vi "AuMT8852B EUT Supported Features Query.vi"(8 "error in (no error)":errorcluster, 11 "VISA session":refnum<visa-resource-name>) -> (0 "error out":errorcluster, 2 "error code":i32, 3 "VISA session out":refnum<visa-resource-name>, 4 "Features":T1)   [LabVIEW 2017]
doc: "Anritsu MT8852B Bluetooth Tester\n\nCauses the tester to query the EUT for a list of supported Bluetooth features.\n\nOUTPUTS\nFeatures - a breakdown of whether or not each Bluetooth feature is present in the EUT."
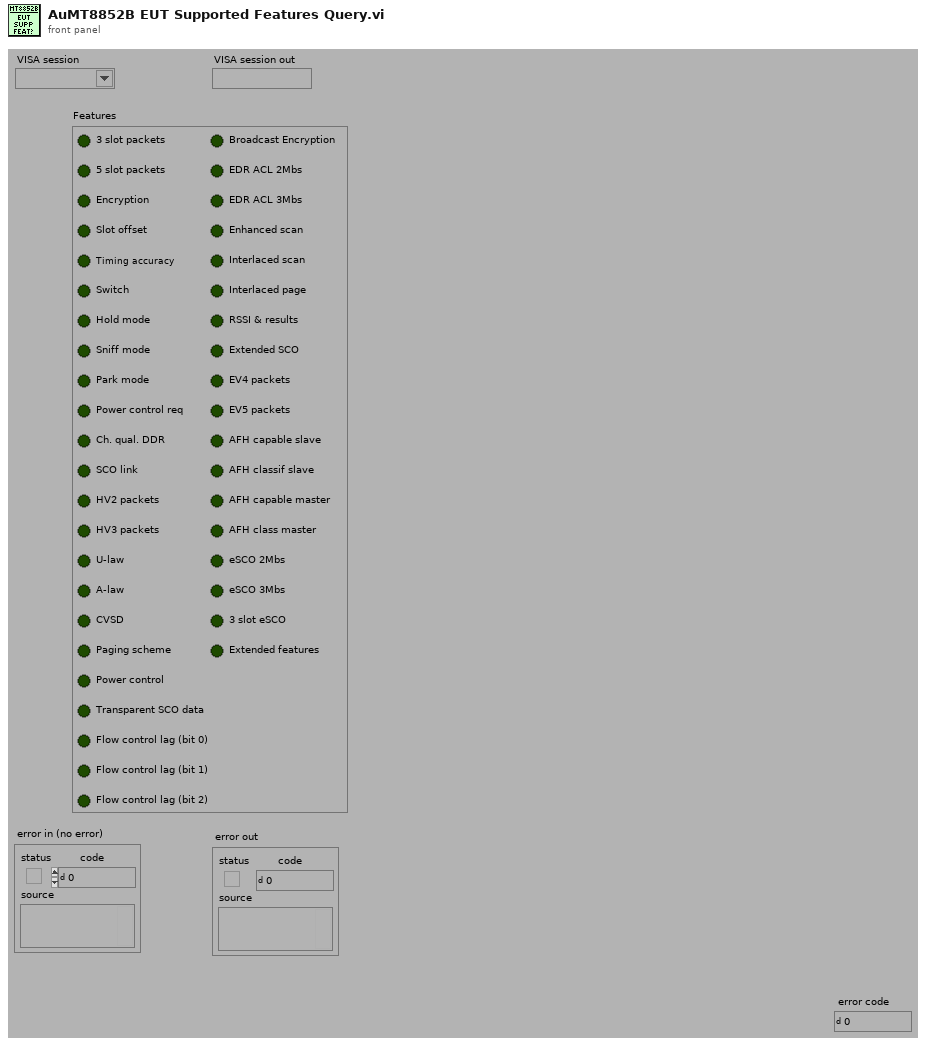
[diagram p1: front panel]
types:
  T1 = cluster{"3 slot packets":bool, "5 slot packets":bool, "Encryption":bool, "Slot offset":bool, "Timing accuracy":bool, "Switch":bool, "Hold mode":bool, "Sniff mode":bool, "Park mode":bool, "Power control req":bool, "Ch. qual. DDR":bool, "SCO link":bool, "HV2 packets":bool, "HV3 packets":bool, "U-law":bool, "A-law":bool, "CVSD":bool, "Paging scheme":bool, "Power control":bool, "Transparent SCO data":bool, "Flow control lag (bit 0)":bool, "Flow control lag (bit 1)":bool, "Flow control lag (bit 2)":bool, "Broadcast Encryption":bool, "EDR ACL 2Mbs":bool, "EDR ACL 3Mbs":bool, "Enhanced scan":bool, "Interlaced scan":bool, "Interlaced page":bool, "RSSI & results":bool, "Extended SCO":bool, "EV4 packets":bool, "EV5 packets":bool, "AFH capable slave":bool, "AFH classif slave":bool, "AFH capable master":bool, "AFH class master":bool, "eSCO 2Mbs":bool, "eSCO 3Mbs":bool, "3 slot eSCO":bool, "Extended features":bool}
  T2 = enum16{"Simulate", "Range check", "Cache", "Query instrument status"}
  T3 = cluster{"Boolean array[0]":bool, "Boolean array[1]":bool, "Boolean array[2]":bool, "Boolean array[3]":bool, "Boolean array[4]":bool, "Boolean array[5]":bool, "Boolean array[6]":bool, "Boolean array[7]":bool, "Boolean array[8]":bool, "Boolean array[9]":bool, "Boolean array[10]":bool, "Boolean array[11]":bool, "Boolean array[12]":bool, "Boolean array[13]":bool, "Boolean array[14]":bool, "Boolean array[15]":bool}
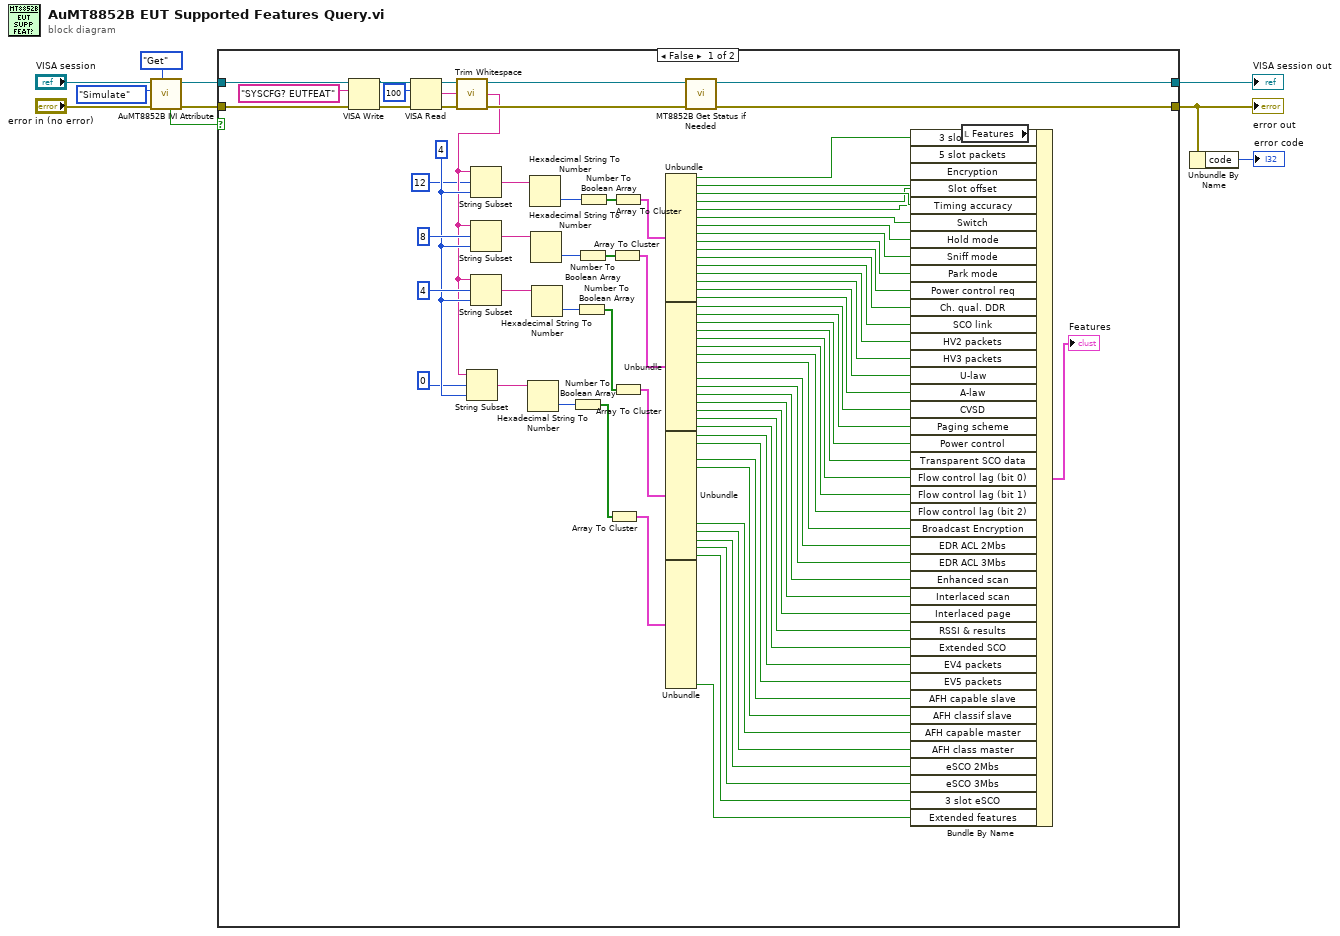
[diagram p0: block diagram]
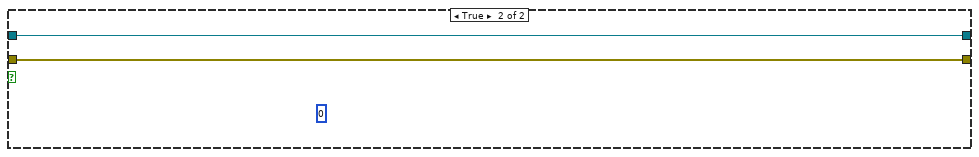
[diagram p2: hidden frame]
diagram:
  n1 = call <instrlib>:"AuMT8852B IVI Attribute.vi"("Set/Get (Set)"=enum16{"Set", "Get"}."Get", "error in (no error)"="error in (no error)", "Flag (Simulate)"=T2."Simulate", "VISA session"="VISA session") -> ("error out"=w7:errorcluster, "VISA session out"=w9:refnum<visa-resource-name>, "Value out"=w3:bool)  [unwired: 5 in]
  n2 = case shown="False" w3 {
    tunnel: [w80 w88] -> w10
    tunnel: [w79 w87] -> w1
    tunnel: w9 -> [w85 w88]
    tunnel: w7 -> [w84 w87]
    frame False {
      w22 = 4 ("length (rest)")
      n3 = VISA Write(VISA resource name=w85, write buffer="SYSCFG? EUTFEAT" ("write buffer (\"\")"), error in (no error)=w84) -> (VISA resource name out=w83:refnum<visa-resource-name>, error out=w82:errorcluster)  [unwired: 1 out]
      n4 = VISA Read(VISA resource name=w83, byte count=u32 100 ("byte count (0)"), error in (no error)=w82) -> (VISA resource name out=w77:refnum<visa-resource-name>, read buffer=w26:string, error out=w78:errorcluster)  [unwired: 1 out]
      n5 = call <vilib>:"Trim Whitespace.vi"("string"=w26) -> ("trimmed string"=w17:string)  [unwired: 1 in]
      n6 = String Subset(string=w17, offset (0)=0, length (rest)=w22) -> (substring=w23:string)
      n7 = String Subset(string=w17, offset (0)=12, length (rest)=w22) -> (substring=w58:string)
      n8 = String Subset(string=w17, offset (0)=8, length (rest)=w22) -> (substring=w54:string)
      n9 = String Subset(string=w17, offset (0)=4, length (rest)=w22) -> (substring=w34:string)
      n10 = Hexadecimal String To Number(string=w23) -> (number=w24:u32)  [unwired: 2 in, 1 out]
      n11 = Hexadecimal String To Number(string=w58) -> (number=w57:u32)  [unwired: 2 in, 1 out]
      n12 = Hexadecimal String To Number(string=w54) -> (number=w53:u32)  [unwired: 2 in, 1 out]
      n13 = Hexadecimal String To Number(string=w34) -> (number=w36:u32)  [unwired: 2 in, 1 out]
      n14 = Number To Boolean Array(number=w24) -> (Boolean array=w20:bool[])
      n15 = Number To Boolean Array(number=w36) -> (Boolean array=w35:bool[])
      n16 = Number To Boolean Array(number=w53) -> (Boolean array=w52:bool[])
      n17 = Number To Boolean Array(number=w57) -> (Boolean array=w56:bool[])
      n18 = Array To Cluster(array=w20) -> (cluster=w19:T3)
      n19 = Array To Cluster(array=w52) -> (cluster=w51:T3)
      n20 = Array To Cluster(array=w56) -> (cluster=w55:T3)
      n21 = Array To Cluster(array=w35) -> (cluster=w33:T3)
      n22 = Unbundle(w55) -> ("Boolean array[0]"=w76:bool, "Boolean array[1]"=w75:bool, "Boolean array[2]"=w74:bool, "Boolean array[3]"=w73:bool, "Boolean array[4]"=w72:bool, "Boolean array[5]"=w71:bool, "Boolean array[6]"=w70:bool, "Boolean array[7]"=w69:bool, "Boolean array[8]"=w68:bool, "Boolean array[9]"=w67:bool, "Boolean array[10]"=w66:bool, "Boolean array[11]"=w65:bool, "Boolean array[12]"=w64:bool, "Boolean array[13]"=w63:bool, "Boolean array[14]"=w62:bool, "Boolean array[15]"=w61:bool)
      n23 = Unbundle(w51) -> ("Boolean array[0]"=w50:bool, "Boolean array[1]"=w49:bool, "Boolean array[2]"=w48:bool, "Boolean array[3]"=w47:bool, "Boolean array[4]"=w46:bool, "Boolean array[5]"=w45:bool, "Boolean array[6]"=w44:bool, "Boolean array[7]"=w25:bool, "Boolean array[9]"=w43:bool, "Boolean array[10]"=w42:bool, "Boolean array[11]"=w41:bool, "Boolean array[12]"=w40:bool, "Boolean array[13]"=w39:bool, "Boolean array[14]"=w38:bool, "Boolean array[15]"=w37:bool)  [unwired: 1 out]
      n24 = Unbundle(w33) -> ("Boolean array[0]"=w32:bool, "Boolean array[1]"=w31:bool, "Boolean array[3]"=w30:bool, "Boolean array[4]"=w29:bool, "Boolean array[11]"=w15:bool, "Boolean array[12]"=w14:bool, "Boolean array[13]"=w13:bool, "Boolean array[14]"=w11:bool, "Boolean array[15]"=w12:bool)  [unwired: 7 out]
      n25 = Unbundle(w19) -> ("Boolean array[15]"=w18:bool)  [unwired: 15 out]
      n26 = call <instrlib>:"MT8852B Get Status if Needed.vi"("error in (no error)"=w78, "VISA session"=w77) -> ("error out"=w79:errorcluster, "VISA session out"=w80:refnum<visa-resource-name>)  [unwired: 8 in]
      n27 = local read "Features"() -> (w59:T1)
      n28 = Bundle By Name(cluster=w59, "3 slot packets"=w76, "5 slot packets"=w75, "Encryption"=w74, "Slot offset"=w73, "Timing accuracy"=w72, "Switch"=w71, "Hold mode"=w70, "Sniff mode"=w69, "Park mode"=w68, "Power control req"=w67, "Ch. qual. DDR"=w66, "SCO link"=w65, "HV2 packets"=w64, "HV3 packets"=w63, "U-law"=w62, "A-law"=w61, "CVSD"=w50, "Paging scheme"=w49, "Power control"=w48, "Transparent SCO data"=w47, "Flow control lag (bit 0)"=w46, "Flow control lag (bit 1)"=w45, "Flow control lag (bit 2)"=w44, "Broadcast Encryption"=w25, "EDR ACL 2Mbs"=w43, "EDR ACL 3Mbs"=w42, "Enhanced scan"=w41, "Interlaced scan"=w40, "Interlaced page"=w39, "RSSI & results"=w38, "Extended SCO"=w37, "EV4 packets"=w32, "EV5 packets"=w31, "AFH capable slave"=w30, "AFH classif slave"=w29, "AFH capable master"=w15, "AFH class master"=w14, "eSCO 2Mbs"=w13, "eSCO 3Mbs"=w11, "3 slot eSCO"=w12, "Extended features"=w18) -> (→"Features":T1)
    }
    frame True {
      (unwired) u8 0
    }
  }
  "error out" <- w1
  "VISA session out" <- w10
  n29 = Unbundle By Name(w1) -> ("code"=→"error code":i32)
